vi "Waveform data class VI - add FFT data.vi"(0 "Waveform data in":refnum<class "Waveform data.lvclass">, 5 "Angles FFT":dbl[](array[numeric]), 7 "displacement FFT":dbl[](array[numeric]), 11 "error in (no error)":errorcluster) -> (4 "Waveform data out":refnum<class "Waveform data.lvclass">, 15 "error out":errorcluster)   [LabVIEW 2010, in "Waveform data.lvclass"]
uses:
  Waveform data.lvclass
  Waveform data.lvclass/Waveform data.ctl
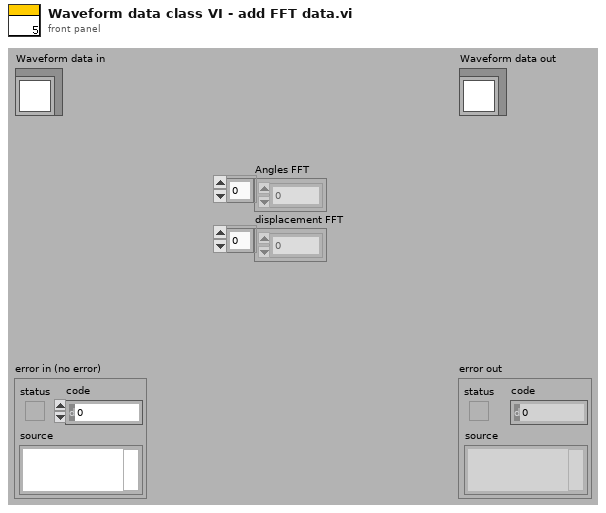
[diagram p1: front panel]
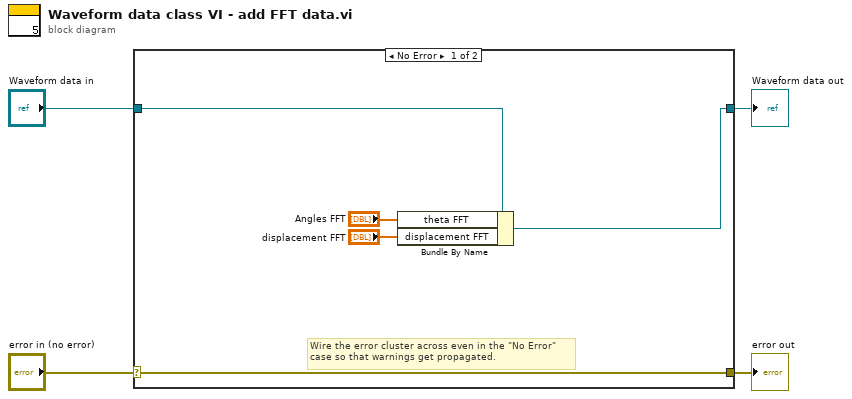
[diagram p0: block diagram]
diagram:
  n1 = case shown="No Error" "error in (no error)" {
    selector: "error in (no error)" -> [w9 w11]
    tunnel: [w9 w11] -> w3
    tunnel: [w7 w10] -> w1
    tunnel: "Waveform data in" -> [w8 w10]
    frame No Error {
      # "Wire the error cluster across even in the \"No Error\"\ncase so that warnings get propagated."
      n2 = Bundle By Name(cluster=w8, "theta FFT"="Angles FFT", "displacement FFT"="displacement FFT") -> (w7:refnum<class "Waveform data.lvclass">)
    }
    frame Error {
    }
  }
  "error out" <- w3
  "Waveform data out" <- w1
